vi "Levels.vi"(9 "Restart":bool, 10 "Mode":enum16{"Slow", "Fast"}(ring), 11 "time signal":waveform(dbl)) -> (1 "Lmin":dbl, 2 "Lpeak":dbl, 3 "Lmax":dbl)   [LabVIEW 2020]
uses:
  <vilib>/Analysis/5stat.llb/RMS (DBL).vi
  <vilib>/Analysis/NI_AALPro.lvlib
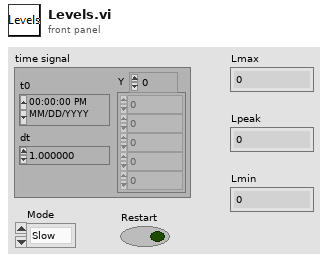
[diagram p1: front panel]
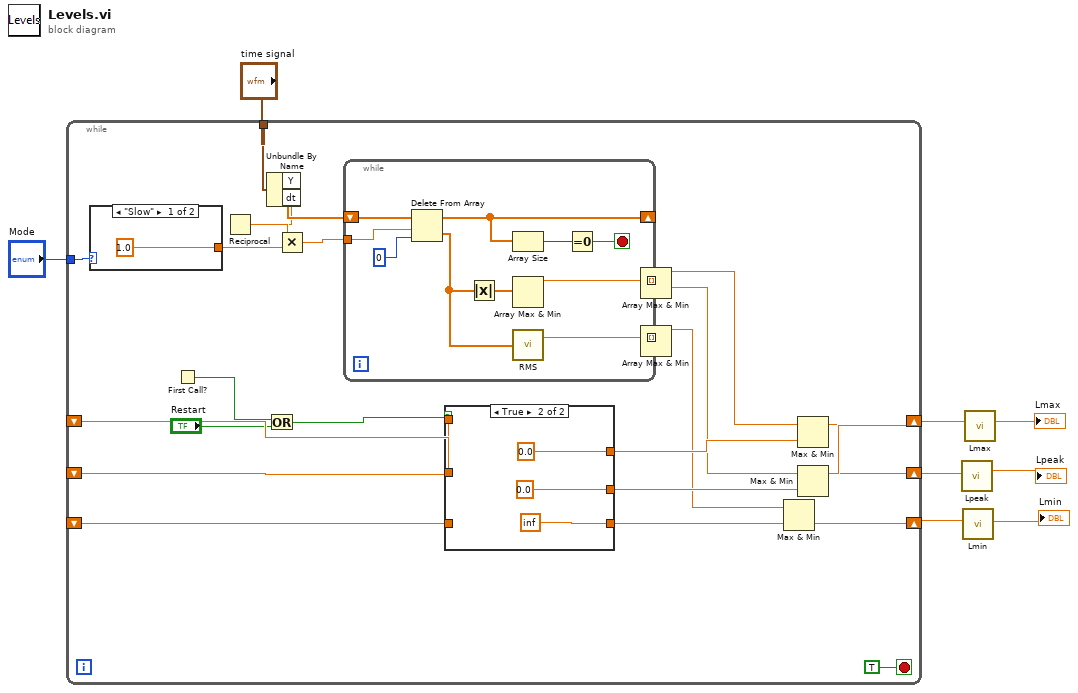
[diagram p0: block diagram]
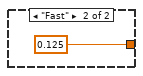
[diagram p2: hidden frame]
diagram:
  n1 = while {
    shift-right: [w27] -> w3
    shift-left: _ -> [w26]
    shift-right: [w9] -> w7
    shift-left: _ -> [w24]
    shift-right: [w18] -> w5
    shift-left: _ -> [w20]
    tunnel: "time signal" -> [w17]
    tunnel: "Mode" -> [w16]
    stop <- TRUE stop-if-true
    n2 = case shown="\"Slow\"" w16 {
      tunnel: [1.0 ("y") 0.125 ("y")] -> w15
      frame "Slow" {
      }
      frame "Fast" {
      }
    }
    n3 = First Call?() -> (First Call?: T/F=w13:bool)
    n4 = Unbundle By Name(w17) -> ("Y"=w31:dbl[], "dt"=w29:dbl)
    n5 = Reciprocal(x=w29) -> (1/x=w30:dbl)
    n6 = Or(x=w13, y="Restart") -> (x .or. y?=w22:bool)
    n7 = Multiply(x=w30, y=w15) -> (x*y=w32:dbl)
    n8 = while {
      shift-right: [w47] -> _
      shift-left: w31 -> [w51]
      tunnel: w32 -> [w50]
      tunnel: [w42] -> w33 mode=indexing
      tunnel: [w43] -> w21 mode=indexing
      stop <- w48 stop-if-true
      n9 = Delete From Array(array=w51, length=w50, index=0) -> (deleted portion=w45:dbl[], array with subset deleted=w47:dbl[])
      n10 = Absolute Value(x=w45) -> (abs(x)=w46:dbl[])
      n11 = Array Size(array=w47) -> (size(s)=w44:i32)
      n12 = Array Max & Min(array=w46) -> (max value=w43:dbl)  [unwired: 3 out]
      n13 = call-poly <vilib>:"RMS.vi"("X"=w45) -> ("rms value"=w42:dbl)  [unwired: 1 out]
      n14 = Equal To 0?(x=w44) -> (x = 0?=w48:bool)
    }
    n15 = case shown="True" w22 {
      tunnel: w26 -> [w38 _]
      tunnel: [w38 0.0] -> w25
      tunnel: w24 -> [w37 _]
      tunnel: [w37 inf] -> w23
      tunnel: w20 -> [w36 _]
      tunnel: [w36 0.0] -> w14
      frame False {
      }
      frame True {
      }
    }
    n16 = Array Max & Min(array=w21) -> (max value=w19:dbl, min value=w11:dbl)  [unwired: 2 out]
    n17 = Array Max & Min(array=w33) -> (max value=w10:dbl)  [unwired: 3 out]
    n18 = Max & Min(x=w10, y=w23) -> (min(x,y)=w9:dbl)  [unwired: 1 out]
    n19 = Max & Min(x=w19, y=w14) -> (max(x,y)=w18:dbl)  [unwired: 1 out]
    n20 = Max & Min(x=w11, y=w25) -> (max(x,y)=w27:dbl)  [unwired: 1 out]
  }
  n21 = call "Lpeak.vi"("Numeric"=w5) -> ("Lpeak"=→"Lpeak":dbl)  [unwired: 10 in]
  n22 = call "Lmin.vi"("Numeric"=w7) -> ("Lmin"=→"Lmin":dbl)  [unwired: 10 in]
  n23 = call "Lmax.vi"("Numeric"=w3) -> ("Lmax"=→"Lmax":dbl)  [unwired: 10 in]
